vi "Get Control Information.vi"(8 "error in (no error)":errorcluster, 11 "Tab in":refnum<class "Tab.lvclass">) -> (0 "error out":errorcluster, 2 "Control Information":string[][](array[string]), 3 "Tab out":refnum<class "Tab.lvclass">)   [LabVIEW 2017, in "Localization.lvlib" / "Tab.lvclass"]
doc: "VI for override that is supposed to do go throgh the process for each control type and pull out the information that is necessary for each control.\n\nChoose Movement Consulting, LLC"
uses:
  Tab.lvclass
  C:/Apps/CMC/OpenSource/Localization/Control Info/Control Info.lvclass
  Control Info/Control Info.lvclass
  Localization.lvlib
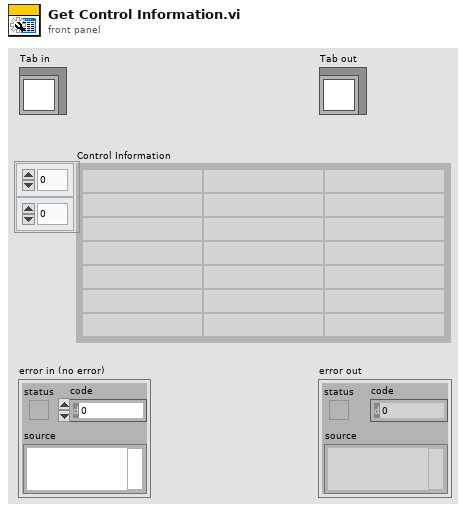
[diagram p1: front panel]
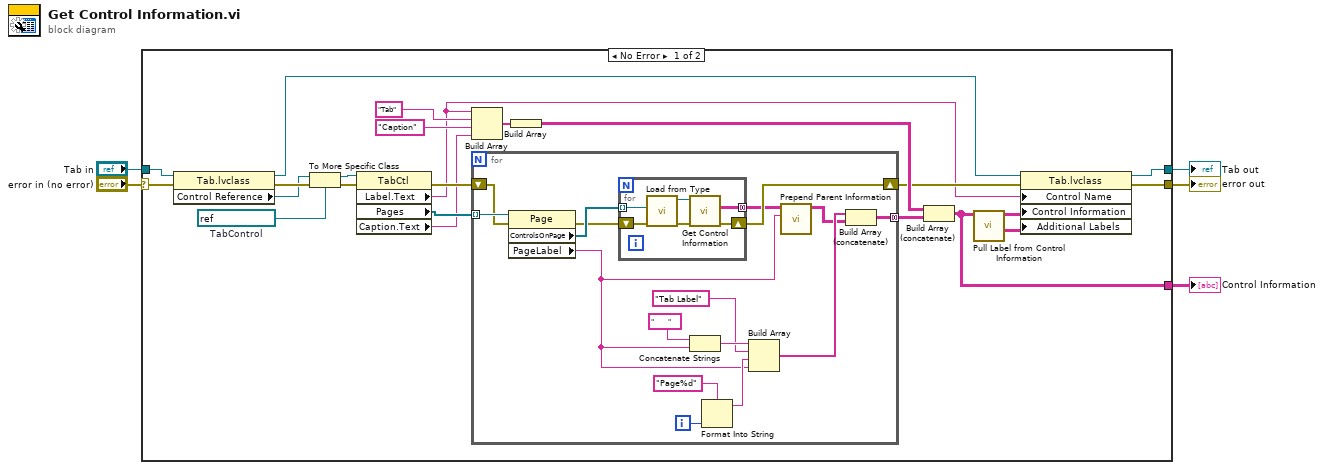
[diagram p0: block diagram]
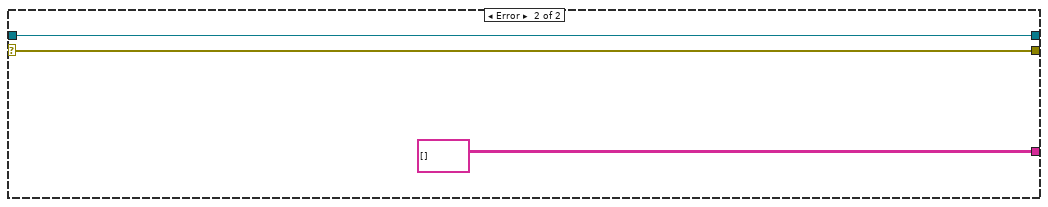
[diagram p2: hidden frame]
diagram:
  n1 = case shown="No Error" "error in (no error)" {
    selector: "error in (no error)" -> [w23 w53]
    tunnel: [w20 w53] -> w1
    tunnel: "Tab in" -> [w22 w52]
    tunnel: [w7 string[][] []] -> w2
    tunnel: [w19 w52] -> w3
    frame No Error {
      w28 = refnum<vi> refnum  # TabControl
      n2 = property class="Tab.lvclass"(reference=w22, error in=w23) -> (reference out=w11:refnum<class "Tab.lvclass">, error out=w24:errorcluster, "Control Reference"=w21:refnum<vi>)
      n3 = To More Specific Class(target class=w28, reference=w21, error in=w24) -> (specific class reference=w27:refnum<vi>, error out=w25:errorcluster)
      n4 = property class="TabCtl"(reference=w27, error in=w25) -> (error out=w14:errorcluster, "Label.Text"=w9:string, "Pages"=w16:refnum<vi>[], "Caption.Text"=w10:string)  [unwired: 1 out]
      n5 = Build Array(w9, "Tab", "Caption", w10) -> (w26:string[])
      n6 = for {
        tunnel: w16 -> [w42] mode=indexing
        tunnel: [w40] -> w12 mode=concatenating
        shift-right: [w44] -> w13
        shift-left: w14 -> [w33]
        i -> [w37]
        n7 = property class="Page"(reference=w42, error in=w33) -> (error out=w32:errorcluster, "ControlsOnPage"=w43:refnum<vi>[], "PageLabel"=w29:string)  [unwired: 1 out]
        n8 = for {
          tunnel: w43 -> [w50] mode=indexing
          shift-right: [w46] -> w44
          shift-left: w32 -> [w49]
          tunnel: [w45] -> w31 mode=concatenating
          n9 = call "Load from Type.vi"("error in (no error)"=w49, "Control Reference"=w50) -> ("error out"=w47:errorcluster, "Control Info out"=w48:refnum<class "Control Info.lvclass">)  [unwired: 8 in]
          n10 = call-dynamic "Get Control Information.vi"("error in (no error)"=w47, "Control Info in"=w48) -> ("error out"=w46:errorcluster, "Control Information"=w45:string[][])  [unwired: 7 in, 1 out]
        }
        n11 = Concatenate Strings("       " ("string"), w29) -> (w41:string)
        n12 = Format Into String(format string="Page%d", w37) -> (resulting string=w36:string)  [unwired: 2 in, 1 out]
        n13 = Build Array(w41, "Tab Label", w36, w29) -> (w34:string[])
        n14 = call "Prepend Parent Information.vi"("Prepend String"=w29, "Control Information in"=w31) -> ("Control Information out"=w30:string[][])  [unwired: 9 in]
        n15 = Build Array (concatenate)(w34, w30) -> (w40:string[][])
      }
      n16 = Build Array(w26) -> (w15:string[][])
      n17 = Build Array (concatenate)(w15, w12) -> (w7:string[][])
      n18 = call "Pull Label from Control Information.vi"("Control Caption Table"=w7) -> ("Additional Labels"=w6:string[][], "Control Information"=w8:string[][])  [unwired: 9 in]
      n19 = property class="Tab.lvclass"(reference=w11, error in=w13, "Control Name"=w9, "Control Information"=w8, "Additional Labels"=w6) -> (reference out=w19:refnum<class "Tab.lvclass">, error out=w20:errorcluster)
    }
    frame Error {
    }
  }
  "error out" <- w1
  "Tab out" <- w3
  "Control Information" <- w2
